vi "TestBINhist_fileContent.vi"() -> ()   [LabVIEW 2020]
uses:
  DBAL/controls/BIN/BINdata.ctl
  DBAL/DBAL-BIN.lvclass
panel:
  out "Array":T1[](array[typedef])
  in  "Numeric Control":i32
  out "XY Graph 2":cluster{"time":dbl[], "min":dbl[]}[](graph)
  out "Numeric 2":i32
  out "Numeric":i32
  out "XY Graph":cluster{"time":dbl[], "min":dbl[]}[](graph)
  out "FileData":T1
  in  "Text Ring":u16(ring)=20 items=["ch0001", "ch0002", "ch0003", "ch0004", "ch0005", "ch0006", "ch0007", "ch0008", "ch0009", "ch0010", "ch0011", "ch0012", "ch0013", "ch0014", "ch0015", "ch0016", "ch0017", "ch0018", "ch0019", "ch0020", "ch0021", "ch0022", "ch0023", "ch0024", "ch0025", "ch0026", "ch0027", "ch0028", "ch0029", "ch0030", "ch0031", "ch0032", "ch0033", "ch0034", "ch0035", "ch0036", "ch0037", "ch0038", "ch0039", "ch0040", "ch0041", "ch0042", "ch0043", "ch0044", "ch0045", "ch0046", "ch0047", "ch0048", "ch0049", "ch0050", "ch0051", "ch0052", "ch0053", "ch0054", "ch0055", "ch0056", "ch0057", "ch0058", "ch0059", "ch0060", "ch0061", "ch0062", "ch0063", "ch0064", "ch0065", "ch0066", "ch0067", "ch0068", "ch0069", "ch0070", "ch0071", "ch0072", "ch0073", "ch0074", "ch0075", "ch0076", "ch0077", "ch0078", "ch0079", "ch0080", "ch0081", "ch0082", "ch0083", "ch0084", "ch0085", "ch0086", "ch0087", "ch0088", "ch0089", "ch0090", "ch0091", "ch0092", "ch0093", "ch0094", "ch0095", "ch0096", "ch0097", "ch0098", "ch0099", "ch0100"]
  out "Left over":i32
  out "Packets":i32
  in  "Path":path=path "C:/Users/Andre/Documents/Sgraph/database/historian/2020-WK21/2020-05-24-PAQ_100mil-002.his"
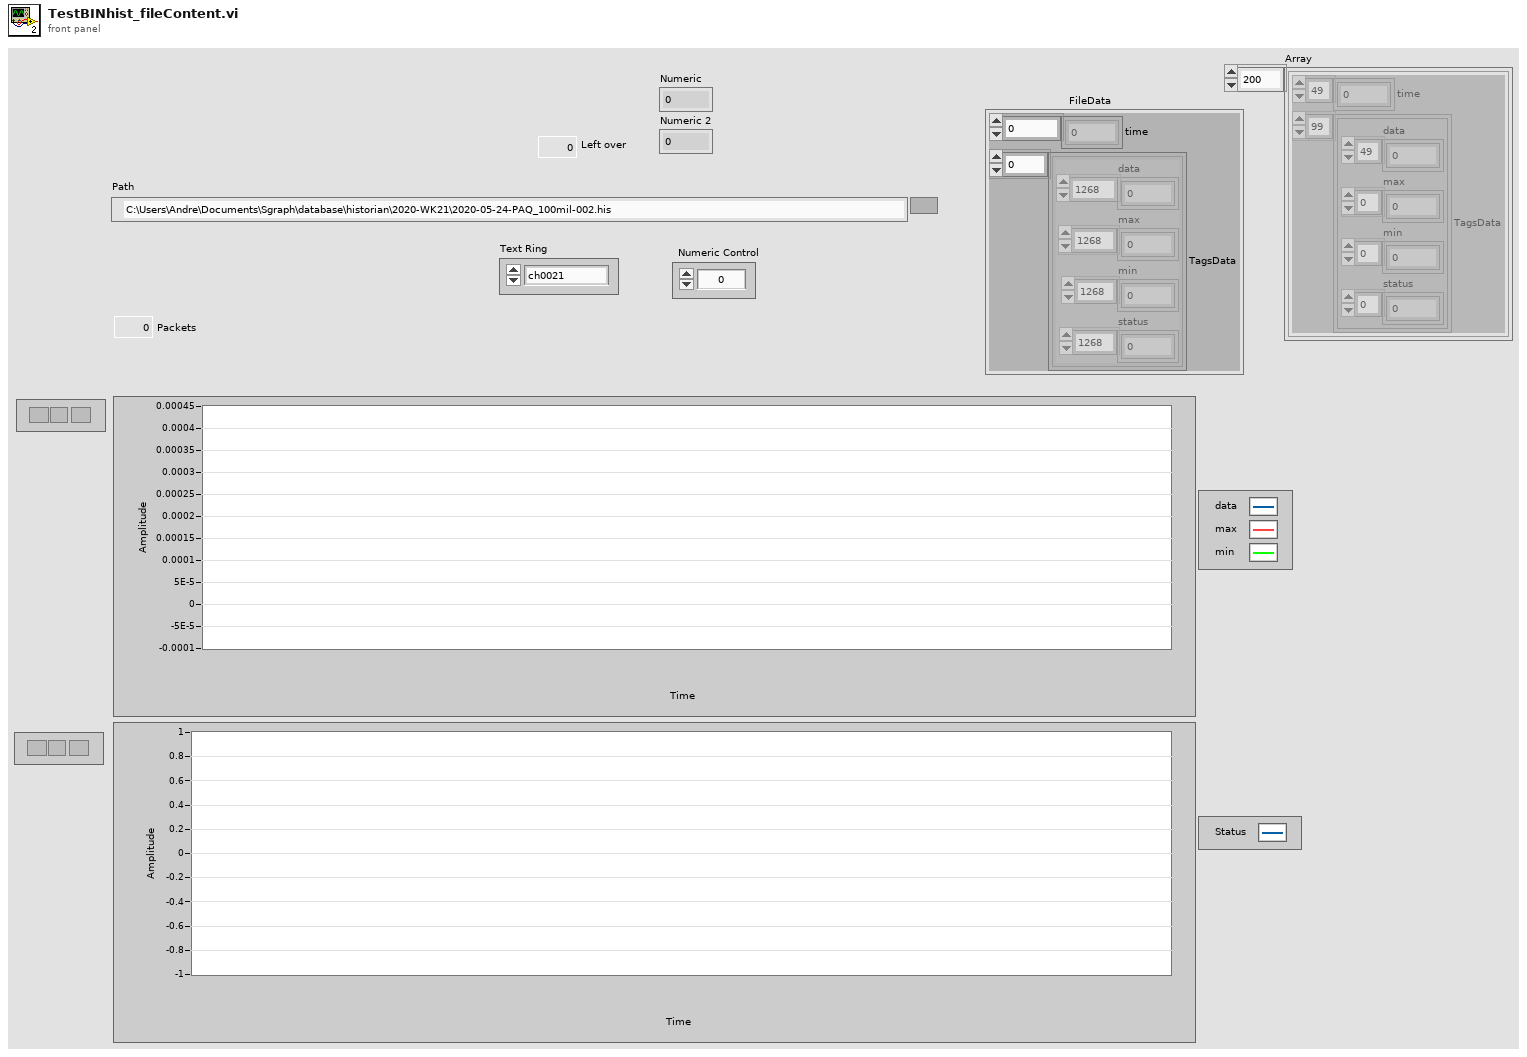
[diagram p1: front panel]
types:
  T1 = typedef "DBAL-BIN.lvclass/BINdata.ctl" = cluster{"time":dbl[], "TagsData":cluster{"data":dbl[], "max":dbl[], "min":dbl[], "status":u32[]}[]}
  T2 = enum16{"big-endian, network order", "native, host order", "little-endian"}
  T3 = cluster{"data":dbl[], "max":dbl[], "min":dbl[], "status":u32[]}[]
  T4 = cluster{"data":dbl[], "max":dbl[], "min":dbl[], "status":u32[]}
  T5 = cluster{"TableName":string, "Data2save":cluster{"TAGs":string[], "time":dbl[], "TagsData":cluster{"data":dbl[], "max":dbl[], "min":dbl[], "status":u32[]}[]}}
  T6 = enum16{"open", "replace", "create", "open or create", "replace or create", "replace or create with confirmation"}
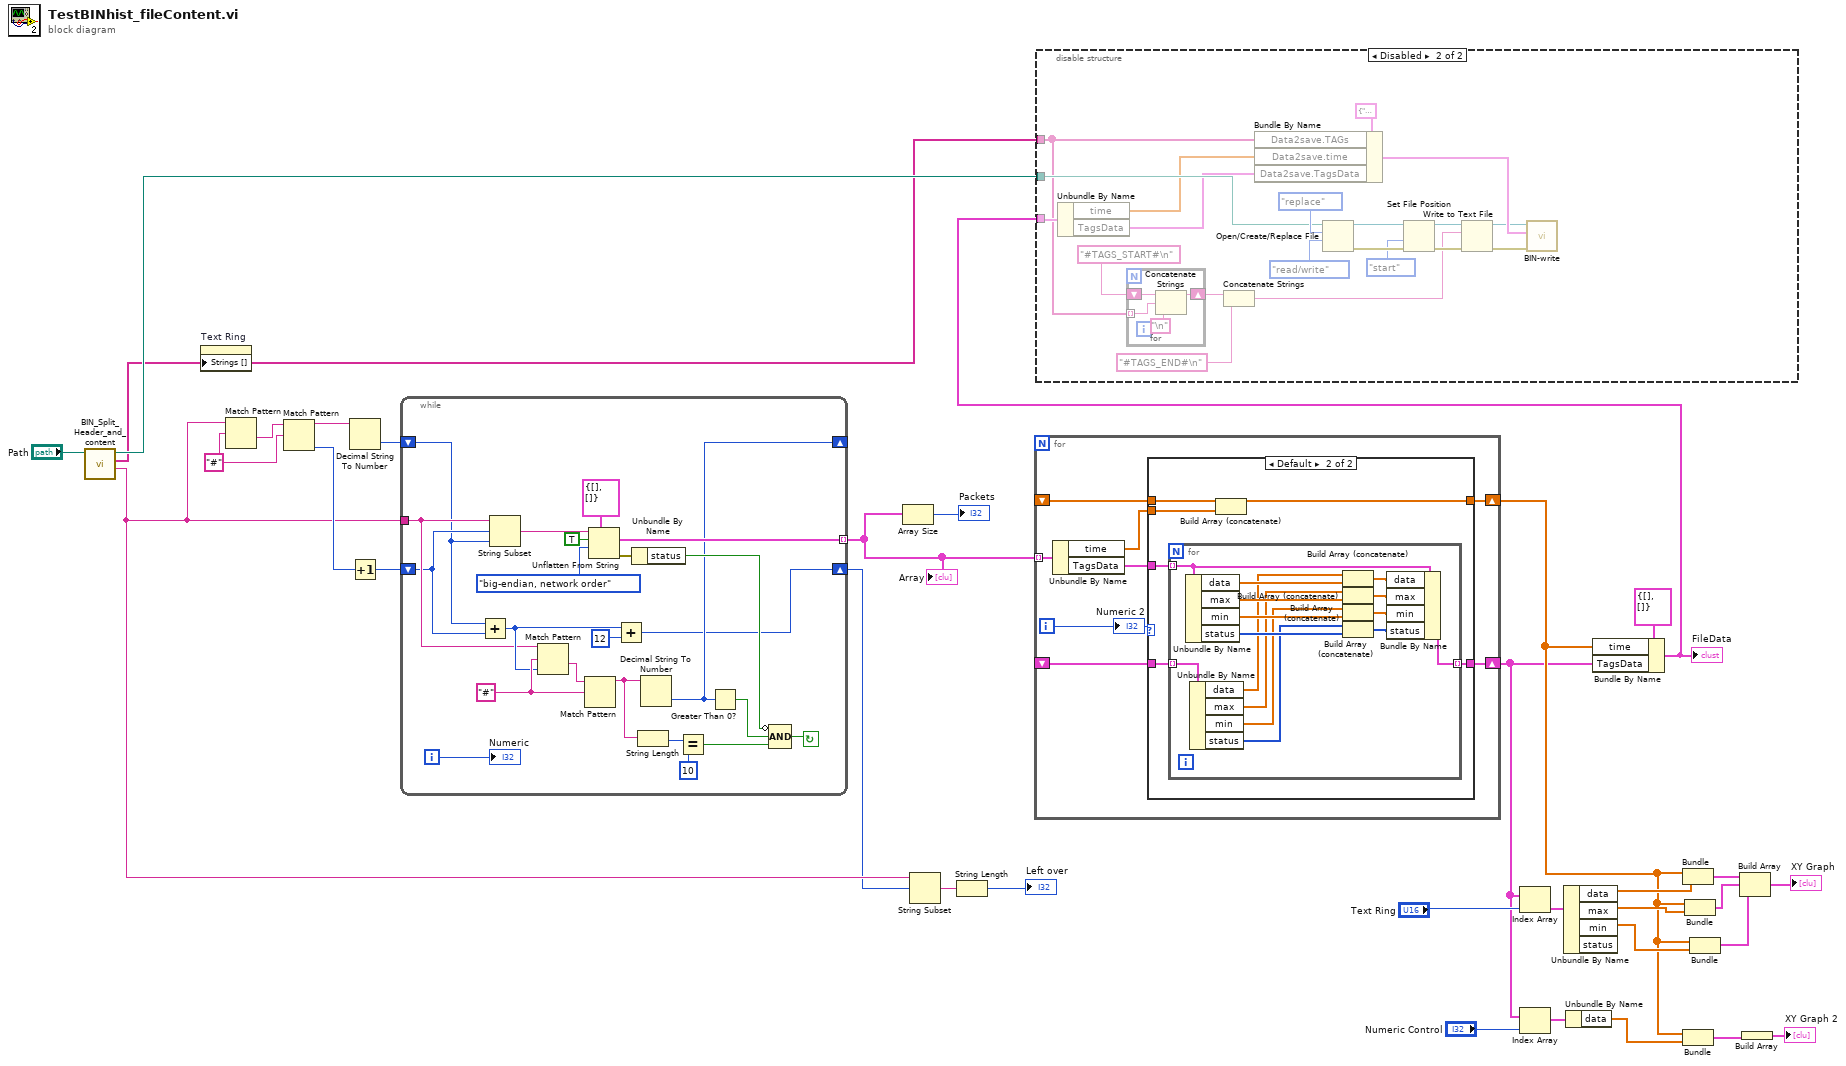
[diagram p0: block diagram]
diagram:
  w30 = "#" ("regular expression")
  n1 = call "BIN_Split_Header_and_content.vi"("Path in"="Path") -> ("Content"=w25:string, "TAGs"=w1:string[], "Path out"=w2:path)  [unwired: 6 in, 2 out]
  n2 = property on="Text Ring" class="Ring (strict)"("Strings []"=w1) -> ()  [unwired: 2 in, 2 out]
  n3 = Match Pattern(string=w25, regular expression=w30) -> (after substring=w31:string)  [unwired: 1 in, 3 out]
  n4 = Match Pattern(string=w31, regular expression=w30) -> (before substring=w33:string, offset past match=w28:i32)  [unwired: 1 in, 2 out]
  n5 = Decimal String To Number(string=w33) -> (number=w32:i32)  [unwired: 2 in, 1 out]
  n6 = Increment(x=w28) -> (x+1=w27:i32)
  n7 = while {
    tunnel: [w53] -> w21 mode=indexing
    shift-right: [w42] -> _
    shift-left: w32 -> [w36]
    shift-right: [w39] -> w24
    shift-left: w27 -> [w37]
    tunnel: w25 -> [w38]
    i -> [w34]
    stop <- w50 continue-if-true
    w52 = "#" ("regular expression")
    n8 = Add(x=w36, y=w37) -> (x+y=w40:i32)
    n9 = String Subset(string=w38, offset (0)=w37, length (rest)=w36) -> (substring=w35:string)
    n10 = Match Pattern(string=w38, regular expression=w52, offset (0)=w40) -> (after substring=w51:string)  [unwired: 3 out]
    n11 = Match Pattern(string=w51, regular expression=w52) -> (before substring=w49:string)  [unwired: 1 in, 3 out]
    n12 = Unflatten From String(type=T1 {"time"=[], "TagsData"=[]} ("BinHistData"), binary string=w35, data includes array or string size? (T)=TRUE, byte order (0:big-endian, network order)=T2."big-endian, network order") -> (value=w53:T1, error out=w44:errorcluster)  [unwired: 1 in, 1 out]
    n13 = Add(x=w40, y=12 ("value")) -> (x+y=w39:i32)
    n14 = Unbundle By Name(w44) -> ("status"=w43:bool)
    n15 = String Length(string=w49) -> (length=w48:i32)
    n16 = Decimal String To Number(string=w49) -> (number=w42:i32)  [unwired: 2 in, 1 out]
    n17 = Equal?(x=w48, y=10) -> (x = y?=w46:bool)
    n18 = Greater Than 0?(x=w42) -> (x > 0?=w45:bool)
    n19 = Compound Arithmetic op=AND(invert w43, w45, w46) -> (w50:bool)
    "Numeric" <- w34
  }
  "Array" <- w21
  n20 = Array Size(array=w21) -> (size(s)=→"Packets":i32)
  n21 = String Subset(string=w25, offset (0)=w24) -> (substring=w23:string)  [unwired: 1 in]
  n22 = String Length(string=w23) -> (length=→"Left over":i32)
  n23 = for {
    tunnel: w21 -> [w57] mode=indexing
    shift-right: [w62] -> w10
    shift-left: _ -> [w64]
    shift-right: [w60] -> w7
    shift-left: _ -> [w58]
    i -> [w61]
    n24 = Unbundle By Name(w57) -> ("time"=w63:dbl[], "TagsData"=w59:T3)
    n25 = case shown="Default" w61 {
      tunnel: w64 -> [_ w72]
      tunnel: w63 -> [w65 w71]
      tunnel: [w65 w70] -> w62
      tunnel: [w66 w67] -> w60
      tunnel: w59 -> [w66 w68]
      tunnel: w58 -> [_ w69]
      frame 0 {
      }
      frame Default {
        n26 = for {
          tunnel: w69 -> [w85] mode=indexing
          tunnel: w68 -> [w87] mode=indexing
          tunnel: [w86] -> w67 mode=indexing
          n27 = Unbundle By Name(w87) -> ("data"=w80:dbl[], "max"=w79:dbl[], "min"=w78:dbl[], "status"=w77:u32[])
          n28 = Unbundle By Name(w85) -> ("data"=w76:dbl[], "max"=w75:dbl[], "min"=w74:dbl[], "status"=w73:u32[])
          n29 = Build Array (concatenate)(w76, w80) -> (w84:dbl[])
          n30 = Build Array (concatenate)(w75, w79) -> (w83:dbl[])
          n31 = Build Array (concatenate)(w74, w78) -> (w82:dbl[])
          n32 = Build Array (concatenate)(w73, w77) -> (w81:u32[])
          n33 = Bundle By Name(cluster=w87, "data"=w84, "max"=w83, "min"=w82, "status"=w81) -> (w86:T4)
        }
        n34 = Build Array (concatenate)(w72, w71) -> (w70:dbl[])
      }
    }
    "Numeric 2" <- w61
  }
  n35 = Index Array(array=w7, index="Text Ring") -> (element=w19:T4)
  n36 = Index Array(array=w7, index="Numeric Control") -> (element=w5:T4)
  n37 = Unbundle By Name(w19) -> ("data"=w13:dbl[], "max"=w12:dbl[], "min"=w11:dbl[])  [unwired: 1 out]
  n38 = Unbundle By Name(w5) -> ("data"=w4:dbl[])
  n39 = Bundle By Name(cluster=T1 {"time"=[], "TagsData"=[]} ("BinHistData"), "time"=w10, "TagsData"=w7) -> (w3:T1)
  "FileData" <- w3
  n40 = disable-structure shown="Disabled" {
    disable-tunnel: w3 -> [_ w100]
    disable-tunnel: w2 -> [_ w102]
    disable-tunnel: w1 -> [_ w89]
    frame Enabled {
    }
    frame Disabled {
      n41 = Unbundle By Name(w100) -> ("time"=w99:dbl[], "TagsData"=w98:T3)
      n42 = for {
        tunnel: w89 -> [w110] mode=indexing
        shift-right: [w109] -> w95
        shift-left: "#TAGS_START#\n" -> [w111]
        n43 = Concatenate Strings(w111, w110, "\n") -> (w109:string)
      }
      n44 = Concatenate Strings(w95, "#TAGS_END#\n") -> (w88:string)
      n45 = Bundle By Name(cluster=T5 {"TableName"="", "Data2save"={"TAGs"=[], "time"=[], "TagsData"=[]}} ("Data in"), "Data2save.TAGs"=w89, "Data2save.time"=w99, "Data2save.TagsData"=w98) -> (w97:T5)
      n46 = Open/Create/Replace File(file path (use dialog)=w102, operation (0:open)=T6."replace", access (0:read/write)=enum16{"read/write", "read-only", "write-only"}."read/write") -> (refnum out=w105:refnum<file>, error out=w104:errorcluster)  [unwired: 3 in, 1 out]
      n47 = Set File Position(refnum=w105, from (0:start)=enum16{"start", "end", "current"}."start", error in=w104) -> (refnum out=w93:refnum<file>, error out=w91:errorcluster)  [unwired: 1 in]
      n48 = Write to Text File(file (use dialog)=w93, text=w88, error in=w91) -> (refnum out=w92:refnum<file>, error out=w90:errorcluster)  [unwired: 1 in, 1 out]
      n49 = call "BIN-write.vi"("error in"=w90, "Data in"=w97, "refnum in"=w92) -> ()  [unwired: 8 in, 1 out]
    }
  }
  n50 = Bundle("time"=w10, "data"=w13) -> (w17:cluster{"time":dbl[], "data":dbl[]})  [unwired: 1 in]
  n51 = Bundle("time"=w10, "data"=w4) -> (w9:cluster{"time":dbl[], "data":dbl[]})  [unwired: 1 in]
  n52 = Bundle("time"=w10, "max"=w12) -> (w16:cluster{"time":dbl[], "max":dbl[]})  [unwired: 1 in]
  n53 = Bundle("time"=w10, "min"=w11) -> (w15:cluster{"time":dbl[], "min":dbl[]})  [unwired: 1 in]
  n54 = Build Array(w17, w16, w15) -> (→"XY Graph":cluster{"time":dbl[], "min":dbl[]}[])
  n55 = Build Array(w9) -> (→"XY Graph 2":cluster{"time":dbl[], "data":dbl[]}[])
